vi "mef.vi"() -> ()   [LabVIEW 2020]
panel:
  in  "stop":bool
  out "caja abierta":bool
  in  "B 12":bool
  in  "B 11":bool
  in  "B 10":bool
  in  "B 9":bool
  in  "B 8":bool
  in  "B 7":bool
  in  "B 6":bool
  in  "B 5":bool
  in  "B 4":bool
  in  "B 3":bool
  in  "B 2":bool
  in  "B 1":bool
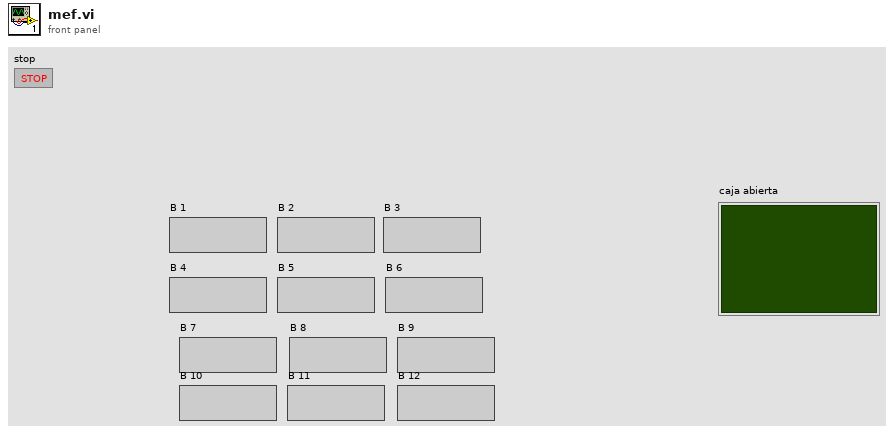
[diagram p1: front panel]
types:
  T1 = enum16{"Estado 0", "Estado 1", "Estado 2", "Estado 3", "Estado 4", "Estado 5", "Estado 6", "Estado 7", "Estado 8", ""}
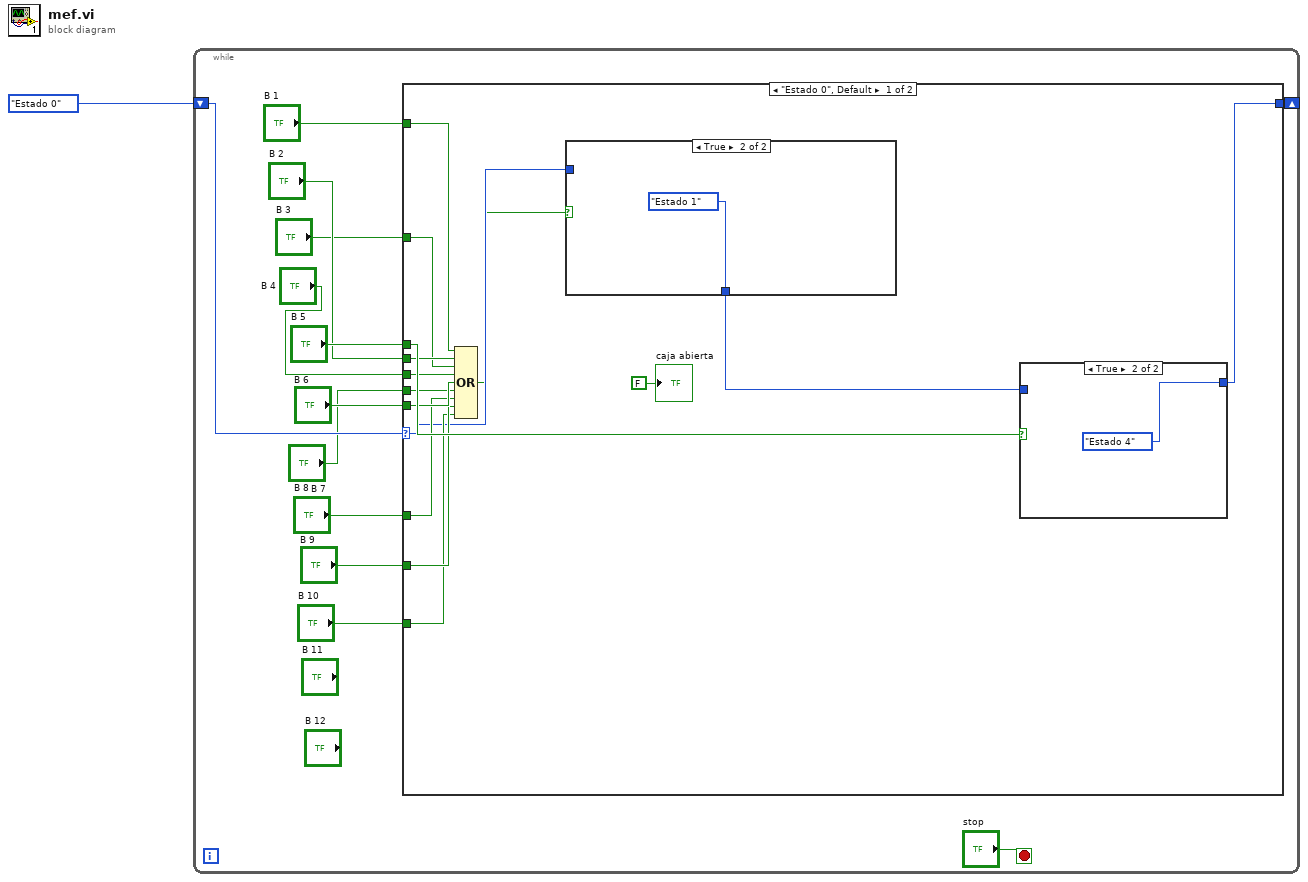
[diagram p0: block diagram]
diagram:
  n1 = while {
    shift-right: [w2] -> _
    shift-left: T1."Estado 0" ("Enum") -> [w13]
    stop <- "stop" stop-if-true
    n2 = case shown="\"Estado 0\", Default" w13 {
      selector: w13 -> [w18 _]
      tunnel: "B 5" -> [w28 _]
      tunnel: "B 1" -> [w27 _]
      tunnel: "B 2" -> [w26 _]
      tunnel: "B 3" -> [w25 _]
      tunnel: "B 4" -> [w24 _]
      tunnel: "B 6" -> [w23 _]
      tunnel: "B 7" -> [w22 _]
      tunnel: "B 8" -> [w21 _]
      tunnel: "B 9" -> [w20 _]
      tunnel: "B 10" -> [w19 _]
      tunnel: [w15 _] -> w2
      frame "Estado 0", Default {
        n3 = Compound Arithmetic op=OR(w27, w26, w25, w24, w23, w22, w21, w20, w19) -> (w16:bool)
        n4 = case shown="True" w16 {
          tunnel: w18 -> [_ _]
          tunnel: [_ T1."Estado 1" ("Enum")] -> w17
          frame False {
          }
          frame True {
          }
        }
        n5 = case shown="True" w28 {
          tunnel: [_ T1."Estado 4" ("Enum")] -> w15
          tunnel: w17 -> [_ _]
          frame False {
          }
          frame True {
          }
        }
        "caja abierta" <- FALSE ("caja abierta")
      }
      frame "Estado 1" {
      }
    }
  }
